vi "Consolidated_Save.vi"(7 "source paths":path[](array[path]), 8 "error in":errorcluster, 9 "Use Consolidated Types":bool, 10 "processed sources":refnum<class "AB_Source.lvclass">[](array[class]), 11 "AB_Targetfile in":refnum<class "AB_Targetfile.lvclass">) -> (0 "error out":errorcluster, 1 "TypeInfo":string, 2 "source destination paths":path[](array[path]), 3 "AB_Targetfile out":refnum<class "AB_Targetfile.lvclass">, 5 "checksums":string[](array[string]))   [LabVIEW 2020, in "AB_Targetfile.lvclass"]
uses:
  <vilib>/AppBuilder/AB_Classes/TargetFile/AB_Targetfile.lvclass
  e:/builds/penguin/labview/branches/2020/dev/dist/vi.lib/AppBuilder/AB_Classes/Build/AB_Build.lvclass
  <vilib>/AppBuilder/AB_Classes/Source/AB_Source.lvclass
  <vilib>/AppBuilder/Engine/AB_Engine_Consolidated_Save_Item_Info.ctl
  <vilib>/AppBuilder/AB_Classes/Build/AB_Build.lvclass
  <vilib>/Utility/lvfile.llb/NI_FileType.lvlib
  <vilib>/AppBuilder/AB_Classes/Destination/AB_Destination.lvclass
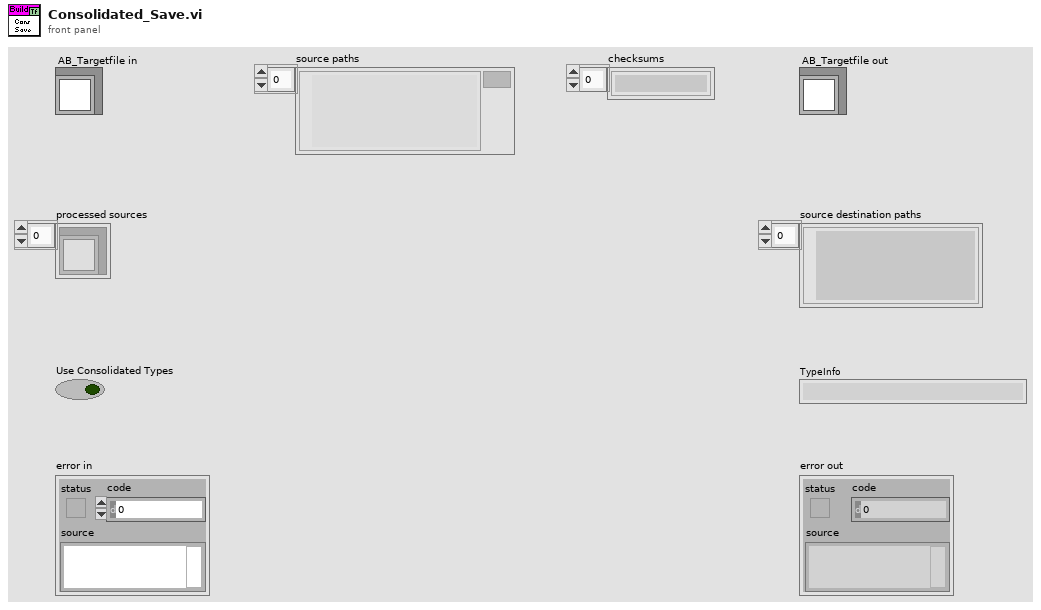
[diagram p1: front panel]
types:
  T1 = typedef "AB_Engine_Consolidated_Save_Item_Info.ctl" = cluster{"Library reference":refnum<vi>, "VI reference":refnum<vi>, "VI save level":i32, "consolidated":bool, "exported":bool}
  T2 = typedef "AB_CopyFiles_Data.ctl" = cluster{"processedItems":T3[]}
  T3 = typedef "AB_Source_Processed_Info.ctl" = cluster{"destPath":path, "buildDelimitedName":string, "sourceIndex":i32, "topLevel":bool}
  T4 = typedef "AB_Build.ctl" = cluster{"buildSpecName":string, "buildSpecDescription":string, "destinations":refnum<class "AB_Destination.lvclass">[], "exclusionOption":T5, "defaultLanguage":string, "supportedLanguages":string[], "excludedDirectories":path[], "buildContext":refnum<vi>, "buildObject":T6, "preview":bool, "programatic":bool, "progressBarEvents":T7, "userLog_Path":path, "preActionID":string, "preAction_Path":path, "postActionID":string, "postAction_Path":path, "eng_checkForBrokenVIs?":bool, "eng_verboseLinkerErrors?":bool, "localDest_Path":path, "targetDest_Path":path, "removeVIObject":u16, "cache":refnum<class "PreviewCache.lvclass">, "use cache":bool, "previewCache_ID":string, "buildCache_ID":string, "eng_TempLocalDest_Path":path, "eng_collectDependencies?":bool, "versionInfo":cluster{"buildVersion":cluster{"major":u16, "minor":u16, "patch":u16, "build":u16}, "autoIncrement":bool}, "eng_enableVIChecksums":bool}
  T5 = typedef "AB_Exclusion_Option.ctl" = cluster{"typedefs":bool, "polymorphicVIs":bool, "unusedLibraryItems":bool, "modifyLibraryFile":bool, "edit-timeDependencies":bool, "inlineVIs":bool, "dependent PPLs":bool, "dependent DLLs":bool}
  T6 = typedef "ItemRef.ctl" = u64
  T7 = typedef "provcom_ProgressBar_Events.ctl" = cluster{"newJob":refnum<user-event>, "newItem":refnum<user-event>, "errorMsg":T8, "cancel":refnum<user-event>}
  T8 = typedef "mxLvBuildError.ctl" = refnum<user-event>
  T9 = typedef "AB_Source.ctl" = cluster{"path":path, "itemID":string, "parentIndex":i32, "sourceInclusion":T10, "destinationIndex":i32, "properties":T11[], "newName":string, "lvfile":bool, "valid":bool, "eng_inBuild":bool, "eng_isNonVILink":bool, "Amalgamation":bool, "Amalgamation Piece":bool, "eng_delimitedName":string, "preventRename":bool}
  T10 = typedef "AB_Source_Inclusion.ctl" = enum16{"IncludeIfReferenced", "Include", "Exclude", "TopLevel"}
  T11 = typedef "AB_Source_Properties.ctl" = cluster{"sourcePropertyType":T12, "value":variant}
  T12 = typedef "AB_Source_Property_Type.ctl" = enum16{"Remove block diagram", "Remove front panel", "Password", "Window has title bar", "Show menu bar", "Show vertical scroll bar", "Show horizontal scroll bar", "Show toolbar", "Show Abort button", "Show fp when called", "Window behavior", "Allow user to close window", "Window run-time position", "Run when opened", "Allow debugging", "Auto error handling", "Generate guard code", "Use stack variables", "Expression folding", "Integer only", "Inline subVI"}
  T13 = typedef "NI_FileType.lvlib/FT_FileTypes.ctl" = enum32{"Invalid file/path", "Unknown type", "Instrument", "Control", "Polymorphic VI", "Project", "Library", "LVClass", "XControl", "XNode", "CIN", "Run-time menu", "Palette menu", "LLB", "Shortcut", "Directory", "Class Private Data Control", "Statechart", "MathScript .m file", "Ladder Diagram", "LVLibp"}
  T14 = typedef "AB_Destination.ctl" = cluster{"destName":string, "path":path, "libraryName":string, "preserveHierarchy":bool, "eng_inBuild":bool, "eng_libraryReference":refnum<vi>, "eng_restictAddToNewLibrary":bool}
  T15 = typedef "AB_Targetfile.ctl" = cluster{"targetfileName":string, "targetfileGUID":string, "enableDebugging":bool, "versionInfo":cluster{"productName":string, "legalCopyright":string, "companyName":string, "internalName":string, "fileDescription":string}, "eng_consolidatedTypeInfo":string, "fastFileFormat":bool, "eng_LEIFBuildData":u32, "versionIndependent":bool}
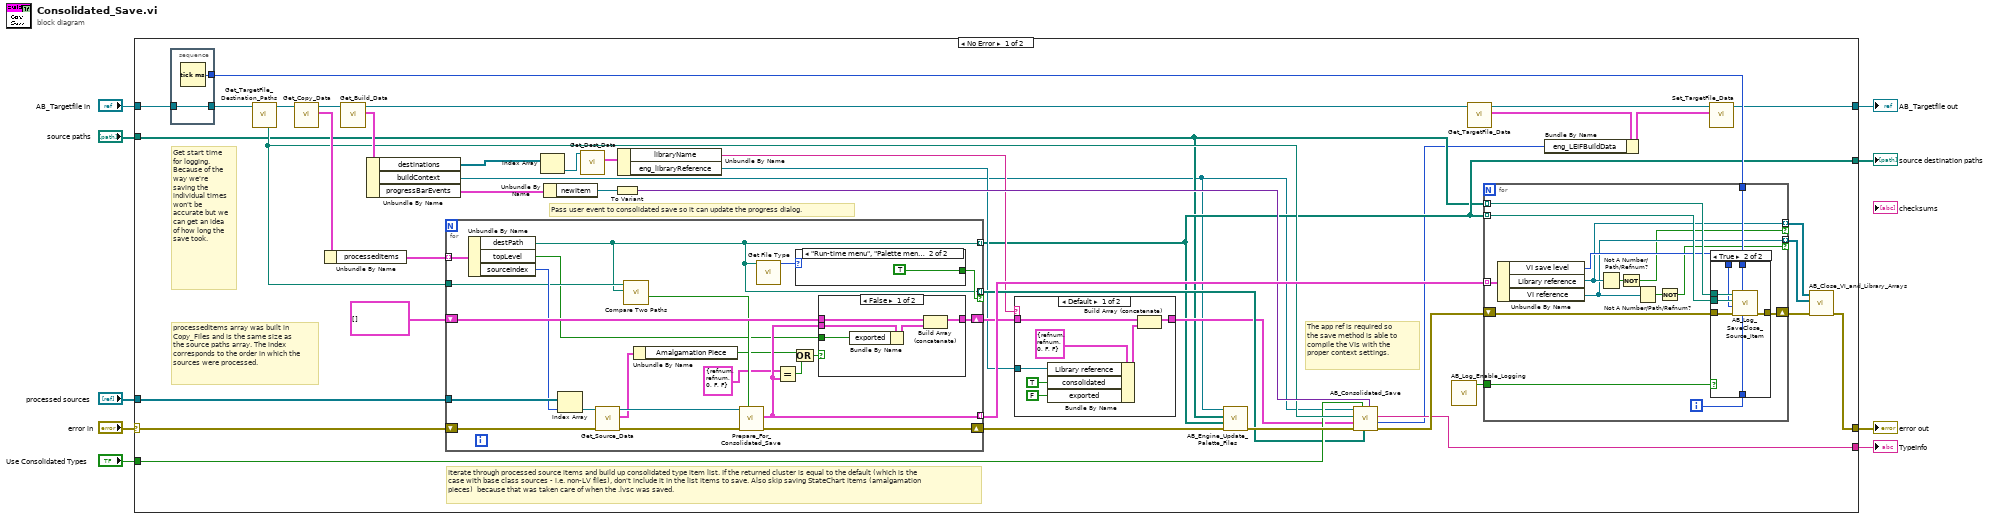
[diagram p0: block diagram]
diagram:
  n1 = case shown="No Error" "error in" {
    selector: "error in" -> [w51 w116]
    tunnel: "processed sources" -> [w46 _]
    tunnel: [w20 _] -> w6
    tunnel: [w45 _] -> w5
    tunnel: "AB_Targetfile in" -> [w44 w115]
    tunnel: [w16 w115] -> w3
    tunnel: [w47 w116] -> w9
    tunnel: "source paths" -> [w19 _]
    tunnel: "Use Consolidated Types" -> [w29 _]
    frame No Error {
      # "Pass user event to consolidated save so it can update the progress dialog."
      # "The app ref is required so the save method is able to compile the VIs with the proper context settings."
      # "processedItems array was built in Copy_Files and is the same size as the source paths array. The index corresponds to the order in which the sources were processed."
      # "Get start time for logging. Because of the way we're saving the individual times won't be accurate but we can get an idea of how long the save took."
      # "Iterate through processed source items and build up consolidated type item list. If the returned cluster is equal to the default (which is the case with base class sources - i.e. non-LV files), don't include it in the list items to save. Also skip saving StateChart items (amalgamation pieces)  because that was taken care of when the .lvsc was saved."
      n2 = stacked-sequence {
        tunnel: w44 -> [w62]
        tunnel: [w62] -> w35
        tunnel: [w61] -> w36
        frame #0 {
          n3 = Tick Count (ms)() -> (millisecond timer value=w61:u32)
        }
      }
      n4 = call <vilib>:"Get_TargetFile_Destination_Paths.vi"("AB_Targetfile in"=w35) -> ("AB_Targetfile out"=w34:refnum<class "AB_Targetfile.lvclass">, "targetfile path"=w30:path)  [unwired: 6 in, 3 out]
      n5 = call <vilib>:"Get_Copy_Data.vi"("AB_Build in"=w34) -> ("copyData"=w39:T2, "AB_Build out"=w40:refnum<class "AB_Targetfile.lvclass">)  [unwired: 8 in, 1 out]
      n6 = Unbundle By Name(w39) -> ("processedItems"=w38:T3[])
      n7 = call <vilib>:"Get_Build_Data.vi"("Class in"=w40) -> ("data"=w41:T4, "Class out"=w17:refnum<class "AB_Targetfile.lvclass">)  [unwired: 8 in, 1 out]
      n8 = Unbundle By Name(w41) -> ("destinations"=w27:refnum<class "AB_Destination.lvclass">[], "buildContext"=w18:refnum<vi>, "progressBarEvents"=w33:T7)
      n9 = for {
        tunnel: w46 -> [w81]
        shift-right: [w79] -> w24
        shift-left: T1[] [] ("Items To Save") -> [w80]
        shift-right: [w84] -> w50
        shift-left: w51 -> [w83]
        tunnel: w38 -> [w78] mode=indexing
        tunnel: [w64] -> w20 mode=indexing
        tunnel: [w77] -> w37 mode=indexing
        tunnel: w30 -> [w75]
        tunnel: [w64] -> w28 mode=indexing if=w65
        n10 = Unbundle By Name(w78) -> ("destPath"=w64:path, "topLevel"=w67:bool, "sourceIndex"=w76:i32)
        n11 = Index Array(array=w81, index=w76) -> (element=w73:refnum<class "AB_Source.lvclass">)
        n12 = call <vilib>:"Get_Source_Data.vi"("error in (no error)"=w83, "Class in"=w73) -> ("error out"=w82:errorcluster, "data"=w71:T9, "Class out"=w72:refnum<class "AB_Source.lvclass">)  [unwired: 7 in]
        n13 = call <vilib>:"Compare Two Paths.vi"("Path 2"=w64, "Path 1"=w75) -> ("Path 2 Relative to Path 1?"=w74:bool)  [unwired: 6 in, 3 out]
        n14 = Unbundle By Name(w71) -> ("Amalgamation Piece"=w70:bool)
        n15 = call-dynamic "Prepare_For_Consolidated_Save.vi"("inside target file"=w74, "error in (no error)"=w82, "AB_Source in"=w72) -> ("error out"=w84:errorcluster, "item_Data"=w77:T1)  [unwired: 6 in, 1 out]
        n16 = call <vilib>:"Get File Type.vi"("path"=w64) -> ("file type"=w66:T13)  [unwired: 8 in, 2 out]
        n17 = Equal?(x=T1 {"Library reference"=refnum, "VI reference"=refnum, "VI save level"=0, "consolidated"=FALSE, "exported"=FALSE}, y=w77) -> (x = y?=w69:bool)
        n18 = Or(x=w70, y=w69) -> (x .or. y?=w68:bool)
        n19 = case shown="\"Run-time menu\", \"Palette menu\"" w66 {
          tunnel: [_ TRUE] -> w65
          frame Default {
          }
          frame "Run-time menu", "Palette menu" {
          }
        }
        n20 = case shown="False" w68 {
          tunnel: w80 -> [w90 w91]
          tunnel: [w89 w91] -> w79
          tunnel: w77 -> [w88 _]
          tunnel: w67 -> [w86 _]
          frame False {
            n21 = Bundle By Name(cluster=w88, "exported"=w86) -> (w87:T1)
            n22 = Build Array (concatenate)(w90, w87) -> (w89:T1[])
          }
          frame True {
          }
        }
      }
      n23 = Index Array(array=w27) -> (element=w26:refnum<class "AB_Destination.lvclass">)  [unwired: 1 in]
      n24 = Unbundle By Name(w33) -> ("newItem"=w32:refnum<user-event>)
      n25 = call <vilib>:"Get_Dest_Data.vi"("Class in"=w26) -> ("destName"=w25:T14)  [unwired: 8 in, 2 out]
      n26 = To Variant(anything=w32) -> (Variant=w31:variant)
      n27 = Unbundle By Name(w25) -> ("libraryName"=w22:string, "eng_libraryReference"=w21:refnum<vi>)
      n28 = case shown="Default" w22 {
        tunnel: [w58 w60] -> w23
        tunnel: w24 -> [w59 w60]
        tunnel: w21 -> [w56 _]
        frame Default {
          n29 = Bundle By Name(cluster=T1 {"Library reference"=refnum, "VI reference"=refnum, "VI save level"=0, "consolidated"=FALSE, "exported"=FALSE}, "Library reference"=w56, "consolidated"=TRUE, "exported"=FALSE) -> (w55:T1)
          n30 = Build Array (concatenate)(w59, w55) -> (w58:T1[])
        }
        frame "" {
          # "This case executes for PPLs because you cannot assign a library to the PPL's main destination."
        }
      }
      n31 = call <vilib>:"AB_Engine_Update_Palette_Files.vi"("error in"=w50, "new paths"=w20, "old paths"=w19, "application reference"=w18) -> ("error out"=w49:errorcluster)  [unwired: 7 in]
      n32 = call <vilib>:"AB_Consolidated_Save.vi"("Progress User Event"=w31, "Run-time and palette menus"=w28, "Use Consolidated Types"=w29, "error in (no error)"=w49, "Items To Save"=w23, "Executable Path"=w30, "app ref in"=w18) -> ("error out"=w52:errorcluster, "LEIF Build Data"=w12:u32, "Consolidated Types"=w45:string)  [unwired: 1 in, 1 out]
      n33 = call <vilib>:"AB_Log_Enable_Logging.vi"() -> ("log?"=w42:bool)  [unwired: 2 in, 9 out]
      n34 = call <vilib>:"Get_TargetFile_Data.vi"("AB_Targetfile in"=w17) -> ("data"=w13:T15, "AB_Targetfile out"=w15:refnum<class "AB_Targetfile.lvclass">)  [unwired: 8 in, 1 out]
      n35 = for {
        tunnel: w36 -> [w103]
        tunnel: w20 -> [w102] mode=indexing
        tunnel: w19 -> [w101] mode=indexing
        shift-right: [w106] -> w48
        shift-left: w52 -> [w105]
        tunnel: w42 -> [w100]
        tunnel: w37 -> [w99] mode=indexing
        tunnel: [w97] -> w10 mode=indexing if=w93
        tunnel: [w96] -> w11 mode=indexing if=w92
        i -> [w104]
        n36 = Unbundle By Name(w99) -> ("VI save level"=w98:i32, "Library reference"=w97:refnum<vi>, "VI reference"=w96:refnum<vi>)
        n37 = Not A Number/Path/Refnum?(number/path/refnum=w97) -> (NaN/Path/Refnum?=w95:bool)
        n38 = Not(x=w95) -> (.not. x?=w93:bool)
        n39 = Not A Number/Path/Refnum?(number/path/refnum=w96) -> (NaN/Path/Refnum?=w94:bool)
        n40 = Not(x=w94) -> (.not. x?=w92:bool)
        n41 = case shown="True" w100 {
          tunnel: w104 -> [_ w112]
          tunnel: w103 -> [_ w111]
          tunnel: w102 -> [_ w110]
          tunnel: w101 -> [_ w109]
          tunnel: [w107 w114] -> w106
          tunnel: w105 -> [w107 w113]
          tunnel: w98 -> [_ w108]
          frame False {
          }
          frame True {
            n42 = call <vilib>:"AB_Log_SaveClose_Source_Item.vi"("index"=w112, "initial time"=w111, "error in (no error)"=w113, "saveLevel"=w108, "destinationPath"=w110, "sourcePath"=w109) -> ("error out"=w114:errorcluster)  [unwired: 5 out]
          }
        }
      }
      n43 = Bundle By Name(cluster=w13, "eng_LEIFBuildData"=w12) -> (w14:T15)
      n44 = call <vilib>:"Set_TargetFile_Data.vi"("data"=w14, "AB_Targetfile in"=w15) -> ("AB_Targetfile out"=w16:refnum<class "AB_Targetfile.lvclass">)  [unwired: 8 in, 1 out]
      n45 = call <vilib>:"AB_Close_VI_and_Library_Arrays.vi"("error in"=w48, "VIs"=w11, "Libraries"=w10) -> ("error out"=w47:errorcluster)  [unwired: 8 in]
    }
    frame Error {
    }
  }
  "error out" <- w9
  "AB_Targetfile out" <- w3
  "source destination paths" <- w6
  "TypeInfo" <- w5
